vi "SBML_File_Parser.vi"(0 "SBML File":path, 2 "SBML Data In":string, 5 "error in (no error)":errorcluster) -> (16 "SBML Data":T2, 19 "error out":errorcluster)   [LabVIEW 2014]
uses:
  Model Information.ctl
panel:
  out "Read SBMLComponents":string
  # "IDs"
  # "Names"
  # "Value"
  # "Information of Parameters"
  # "Information of Species"
  # "IDs"
  # "Names"
  # "Initial Amount"
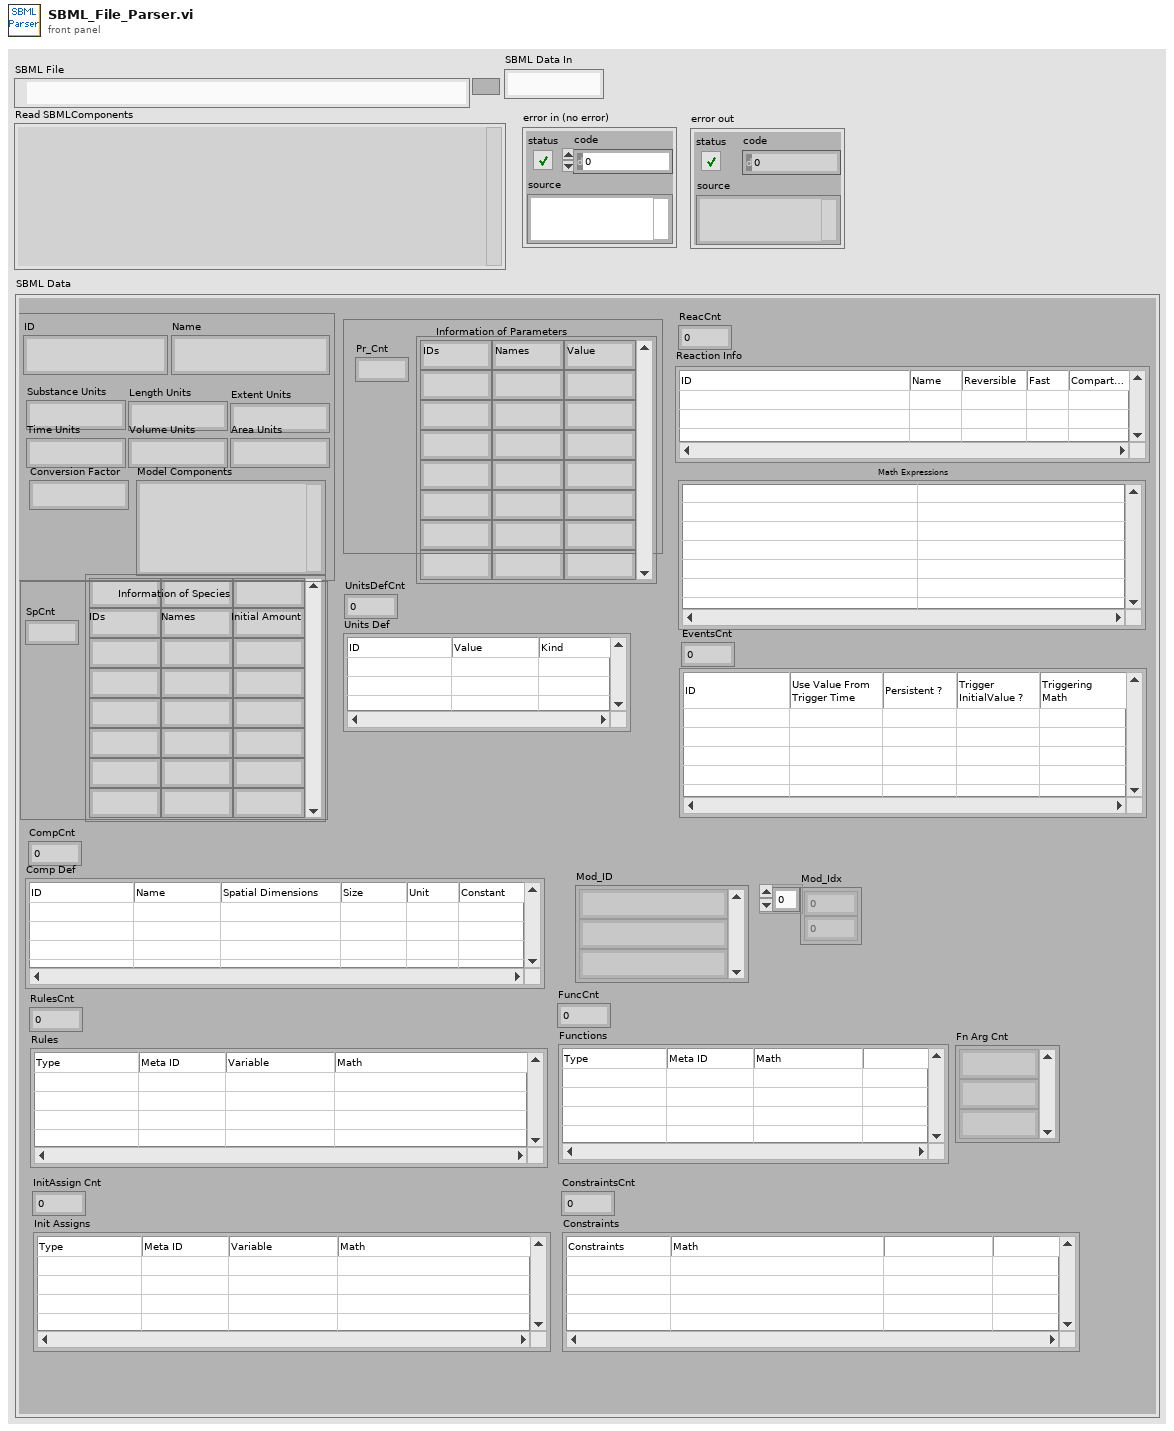
[diagram p1: front panel]
types:
  T1 = typedef "Model Information.ctl" = cluster{"ID":string, "Name":string, "Substance Units":string, "Time Units":string, "Volume Units":string, "Area Units":string, "Length Units":string, "Extent Units":string, "Conversion Factor":string, "Model Components":string}
  T2 = cluster{"Model Info":T1, "SpCnt":i32, "Species Info":string[][], "Pr_Cnt":i32, "Parameter info":string[][], "ReacCnt":i32, "Reaction Info":string[][], "Math Expressions":string[][], "EventsCnt":i32, "Event Info":string[][], "UnitsDefCnt":i32, "Units Def":string[][], "CompCnt":i32, "Comp Def":string[][], "Mod_ID":string[], "Mod_Idx":i32[], "RulesCnt":i32, "Rules":string[][], "FuncCnt":i32, "Functions":string[][], "InitAssign Cnt":i32, "Init Assigns":string[][], "ConstraintsCnt":i32, "Constraints":string[][], "Fn Arg Cnt":string[]}
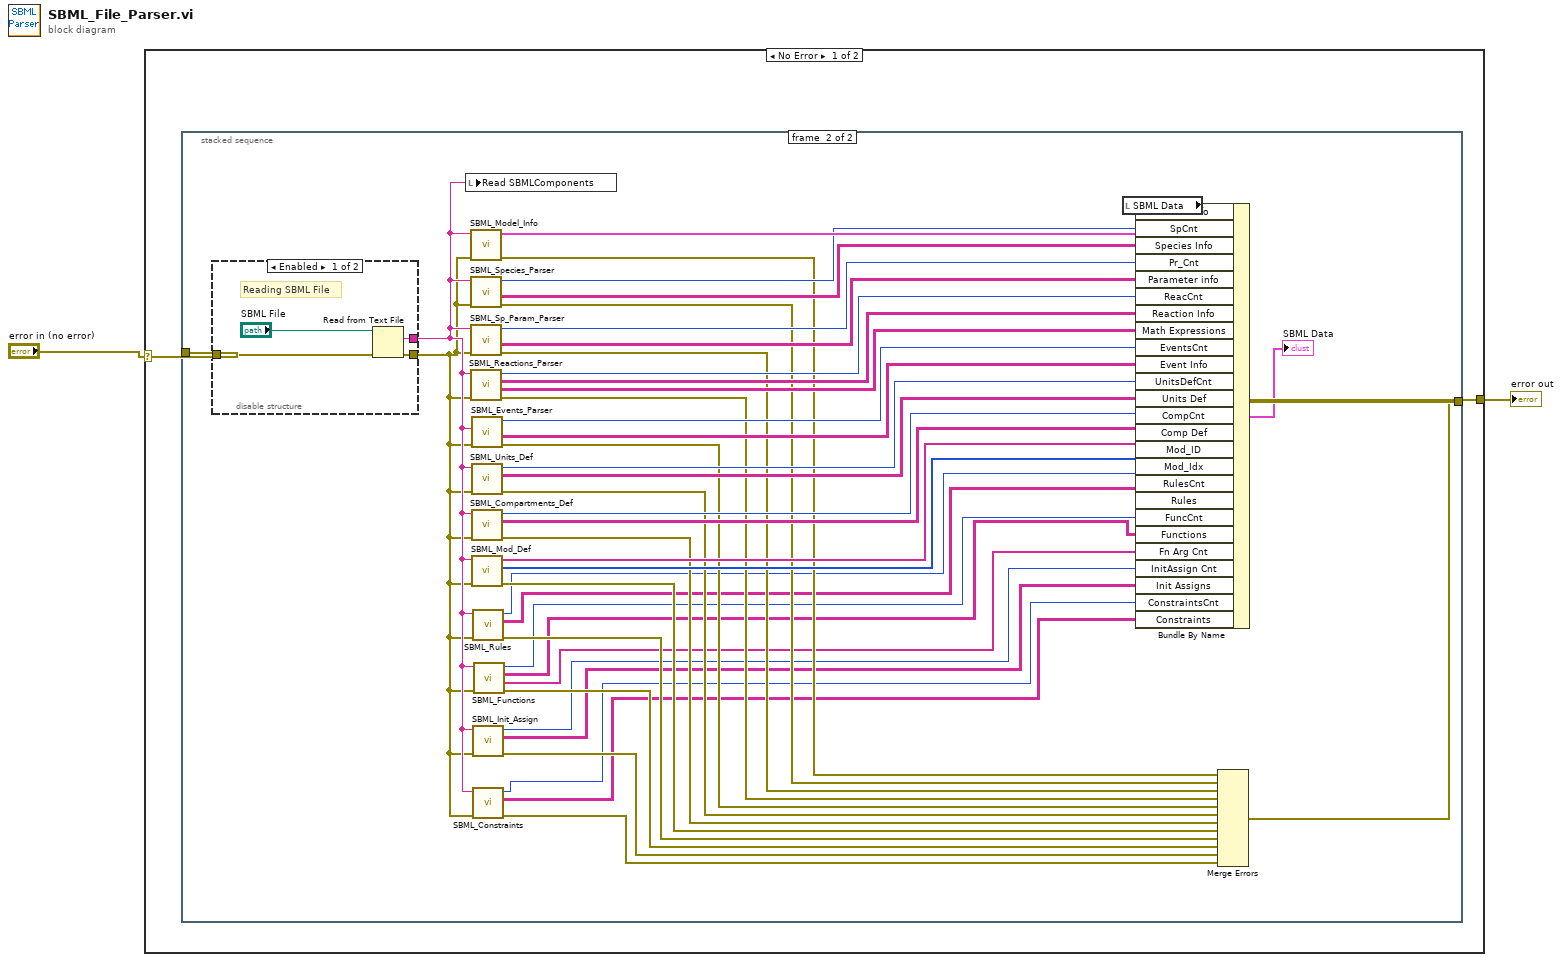
[diagram p0: block diagram]
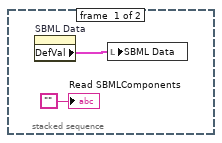
[diagram p2: hidden frame]
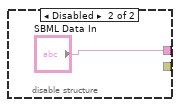
[diagram p3: hidden frame]
diagram:
  n1 = case shown="No Error" "error in (no error)" {
    selector: "error in (no error)" -> [w4 w55]
    tunnel: [w3 w55] -> w1
    frame No Error {
      n2 = stacked-sequence {
        tunnel: w4 -> [_ w49]
        tunnel: [_ w22] -> w3
        frame #0 {
          n3 = property on="SBML Data" class="Clust (strict)"() -> ("DefVal"=w5:T2)  [unwired: 2 in, 2 out]
          n4 = local write "SBML Data"(w5) -> ()
          "Read SBMLComponents" <- ""
        }
        frame #1 {
          n5 = disable-structure shown="Enabled" {
            disable-tunnel: w49 -> [w53 _]
            disable-tunnel: [w51 "SBML Data In"] -> w12
            disable-tunnel: [w50 _] -> w11
            frame Enabled {
              # "Reading SBML File"
              n6 = Read from Text File(file (use dialog)="SBML File", error in=w53) -> (text=w51:string, error out=w50:errorcluster)  [unwired: 2 in, 2 out]
            }
            frame Disabled {
            }
          }
          n7 = local write "Read SBMLComponents"(w12) -> ()
          n8 = call "SBML_Model_Info.vi"("error in (no error)"=w11, "Input SBML File"=w12) -> ("error out"=w30:errorcluster, "Model Information"=w46:T1)  [unwired: 8 in]
          n9 = call "SBML_Species_Parser.vi"("error in (no error)"=w11, "Input SBML File"=w12) -> ("error out"=w29:errorcluster, "Species Info"=w44:string[][], "Sp_Cnt"=w45:i32)  [unwired: 7 in]
          n10 = call "SBML_Sp_Param_Parser.vi"("error in (no error)"=w11, "Input SBML File"=w12) -> ("error out"=w28:errorcluster, "Param Info"=w42:string[][], "Pr_Cnt"=w43:i32)  [unwired: 7 in]
          n11 = call "SBML_Reactions_Parser.vi"("error in (no error)"=w11, "Input SBML File"=w12) -> ("error out"=w27:errorcluster, "Reaction Math"=w39:string[][], "Reaction Info"=w40:string[][], "Reac_cnt"=w41:i32)  [unwired: 4 in]
          n12 = call "SBML_Events_Parser.vi"("error in (no error)"=w11, "Input SBML File"=w12) -> ("error out"=w26:errorcluster, "Event Info"=w37:string[][], "Event_cnt"=w38:i32)  [unwired: 5 in]
          n13 = call "SBML_Units_Def.vi"("error in (no error)"=w11, "Input SBML File"=w12) -> ("error out"=w25:errorcluster, "Units Definition"=w35:string[][], "Units_Cnt"=w36:i32)  [unwired: 7 in]
          n14 = call "SBML_Compartments_Def.vi"("error in (no error)"=w11, "Input SBML File"=w12) -> ("error out"=w24:errorcluster, "Compartments Definition"=w33:string[][], "Compartments_Cnt"=w34:i32)  [unwired: 7 in]
          n15 = call "SBML_Mod_Def.vi"("error in (no error)"=w11, "Input SBML File"=w12) -> ("error out"=w23:errorcluster, "Mod_Idx"=w31:i32[], "Mod_ID"=w32:string[])  [unwired: 7 in]
          n16 = call "SBML_Rules.vi"("error in (no error)"=w11, "Input SBML File"=w12) -> ("error out"=w21:errorcluster, "Rules"=w19:string[][], "RulesCnt"=w20:i32)  [unwired: 7 in]
          n17 = call "SBML_Init_Assign.vi"("error in (no error)"=w11, "Input SBML File"=w12) -> ("error out"=w15:errorcluster, "Initial Assignments"=w13:string[][], "InitAssignCnt"=w14:i32)  [unwired: 7 in]
          n18 = call "SBML_Constraints.vi"("error in (no error)"=w11, "Input SBML File"=w12) -> ("error out"=w8:errorcluster, "Constraints"=w9:string[][], "ConstraintsCnt"=w10:i32)  [unwired: 7 in]
          n19 = call "SBML_Functions.vi"("error in (no error)"=w11, "Input SBML File"=w12) -> ("error out"=w18:errorcluster, "Fn Arg Cnt"=w7:string[], "Functions"=w16:string[][], "FuncCnt"=w17:i32)  [unwired: 6 in]
          n20 = local read "SBML Data"() -> (w47:T2)
          n21 = Bundle By Name(cluster=w47, "Model Info"=w46, "SpCnt"=w45, "Species Info"=w44, "Pr_Cnt"=w43, "Parameter info"=w42, "ReacCnt"=w41, "Reaction Info"=w40, "Math Expressions"=w39, "EventsCnt"=w38, "Event Info"=w37, "UnitsDefCnt"=w36, "Units Def"=w35, "CompCnt"=w34, "Comp Def"=w33, "Mod_ID"=w32, "Mod_Idx"=w31, "RulesCnt"=w20, "Rules"=w19, "FuncCnt"=w17, "Functions"=w16, "Fn Arg Cnt"=w7, "InitAssign Cnt"=w14, "Init Assigns"=w13, "ConstraintsCnt"=w10, "Constraints"=w9) -> (→"SBML Data":T2)
          n22 = Merge Errors(w30, w29, w28, w27, w26, w25, w24, w23, w21, w18, w15, w8) -> (w22:errorcluster)
        }
      }
    }
    frame Error {
    }
  }
  "error out" <- w1
